vi "DFD FXP Simulation with State.vi"   [LabVIEW 2017, in "NI_DigFilterLicensed.lvlib"]
doc: "Simulates the filtering process with initial internal states and generates the filtering statistics report for a fixed-point filter. The data type you wire to the <B>signal in</B> input determines the polymorphic instance to use."
uses:
  <vilib>/addons/Digital Filter Design/NI_DigFilterLicensed.lvlib
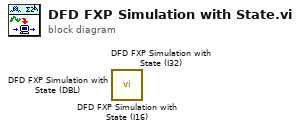
[diagram p0: block diagram]
diagram:
  n1 = call <vilib>:"DFD FXP Simulation with State (I16).vi"() -> ()  [unwired: 7 in, 5 out]
  n2 = call <vilib>:"DFD FXP Simulation with State (I32).vi"() -> ()  [unwired: 7 in, 5 out]
  n3 = call <vilib>:"DFD FXP Simulation with State (DBL).vi"() -> ()  [unwired: 7 in, 5 out]
